vi "Configure Hold.vi"(8 "error in (no error)":errorcluster, 10 "Hold Mode (0)":i8(ring) items=["OFF", "ON", "TOGGLE"], 11 "VISA resource name":refnum<visa-resource-name>) -> (0 "error out":errorcluster, 3 "VISA resource name out":refnum<visa-resource-name>)   [LabVIEW 2017, in "BK Precision 1823A.lvlib"]
doc: "This VI controls the hold function of the counter. For <b>Hold Mode</b>, Input integer 0 for OFF, 1 for ON, and 2 for TOGGLE."
uses:
  BK Precision 1823A.lvlib
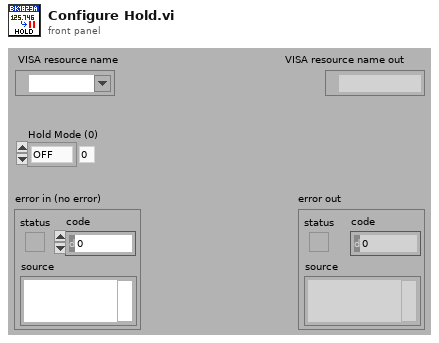
[diagram p1: front panel]
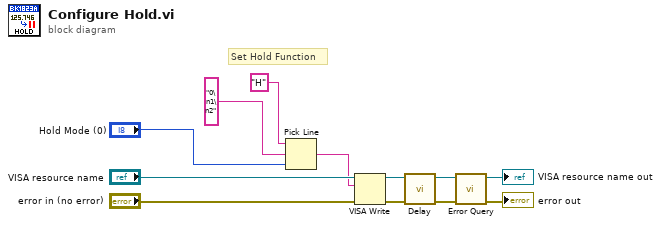
[diagram p0: block diagram]
diagram:
  # "Set Hold Function"
  n1 = Pick Line(string ("")="H", multi-line string="0\n1\n2", line index="Hold Mode (0)") -> (output string=w6:string)
  n2 = VISA Write(VISA resource name="VISA resource name", write buffer=w6, error in (no error)="error in (no error)") -> (VISA resource name out=w4:refnum<visa-resource-name>, error out=w1:errorcluster)  [unwired: 1 out]
  n3 = call "Delay.vi"("error in (no error)"=w1, "VISA resource name"=w4) -> ("error out"=w2:errorcluster, "VISA resource name out"=w3:refnum<visa-resource-name>)  [unwired: 8 in]
  n4 = call "Error Query.vi"("error in (no error)"=w2, "VISA resource name"=w3) -> ("error out"=→"error out":errorcluster, "VISA resource name out"=→"VISA resource name out":refnum<visa-resource-name>)  [unwired: 8 in]
